vi "CRC for DM3-10A.vi"(0 "CMD":u8[](array[numeric]), 1 "error in (no error)":errorcluster caption="错误输入（无错误）") -> (2 "CRC":u16 format="%.0x", 3 "CRCHi":u8 format="%.0x", 4 "CRCLo":u8 format="%.0x", 5 "error out":errorcluster caption="错误输出")   [LabVIEW 2015]
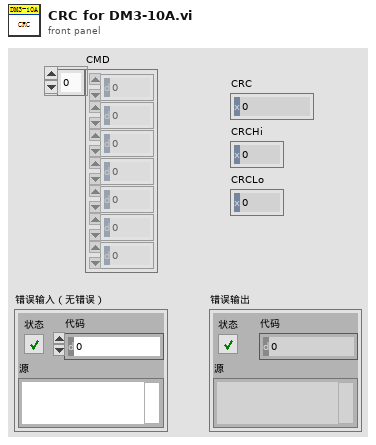
[diagram p1: front panel]
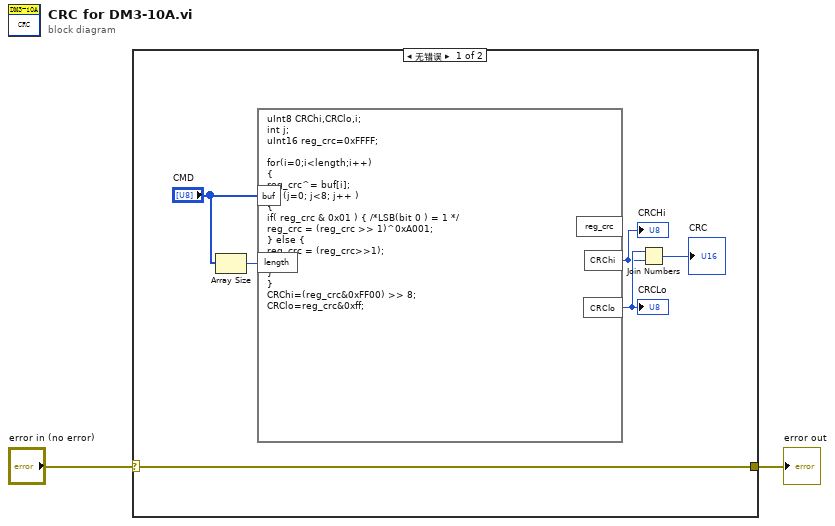
[diagram p0: block diagram]
diagram:
  n1 = case shown="无错误" "error in (no error)" {
    selector: "error in (no error)" -> [w3 w9]
    tunnel: [w3 w9] -> w1
    frame No Error {
      n2 = Array Size(array="CMD") -> (size(s)=w8:i32)
      n3 = formula code="uInt8 CRChi,CRClo,i;\nint j; \nuInt16 reg_crc=0xFFFF; \n \nfor(i=0;i<length;i++) \n{ \nreg_crc^= buf[i]; \nfor (j=0; j<8; j++ ) \n{ \nif( reg_crc & 0x01 ) { /*LSB(bit 0 ) = 1 */ \nreg_crc = (reg_crc >> 1)^0xA001; \n} else { \nreg_crc = (reg_crc>>1); \n} \n} \n} \nCRChi=(reg_crc&0xFF00) >> 8;\nCRClo=reg_crc&0xff;"("buf"="CMD", "length"=w8) -> ("CRChi"=w5:u8, "CRClo"=w6:u8)  [unwired: 1 out]
      "CRCLo" <- w6
      "CRCHi" <- w5
      n4 = Join Numbers(hi=w6, lo=w5) -> ((hi.lo)=→"CRC":u16)
    }
    frame Error {
    }
  }
  "error out" <- w1
